vi "Point-in-Quad test (axis-aligned).vi"(1 "Point":sgl[](array[numeric]), 2 "Quad":T1) -> (0 "Point is inside quad":bool)   [LabVIEW 2014]
uses:
  Typedefs/Quad.ctl
  Typedefs/Quadplane enum.ctl
panel:
  # "PN 17/01/2015, 25/03/2015"
  # "Vertices"
  # "Edges"
  # "Unit normal"
  # "Plane ident."
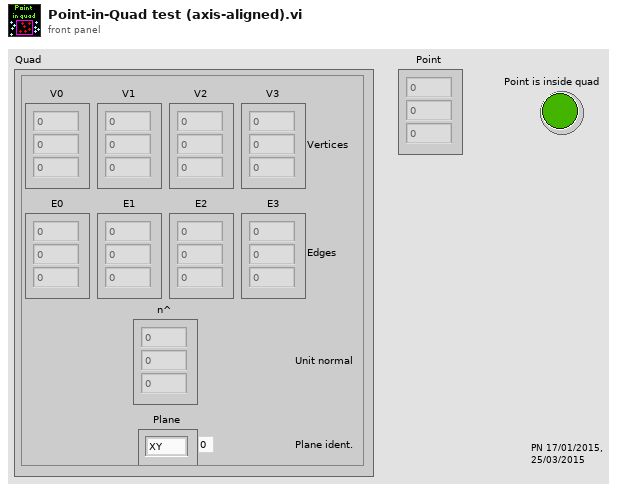
[diagram p1: front panel]
types:
  T1 = typedef "Quad.ctl" = cluster{"V0":sgl[], "V1":sgl[], "V2":sgl[], "V3":sgl[], "E0":sgl[], "E1":sgl[], "E2":sgl[], "E3":sgl[], "n^":sgl[], "Plane":T2}
  T2 = typedef "Quadplane enum.ctl" = enum8{"XY", "XZ", "YZ", "-XY", "-XZ", "-YZ"}
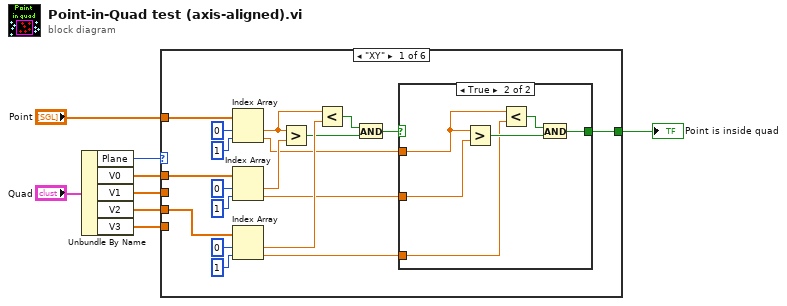
[diagram p0: block diagram]
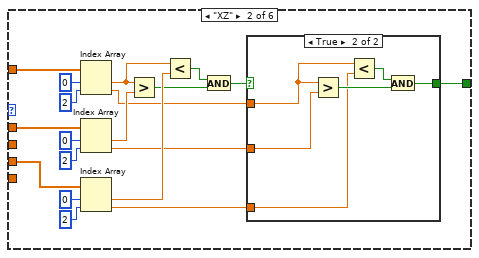
[diagram p3: hidden frame]
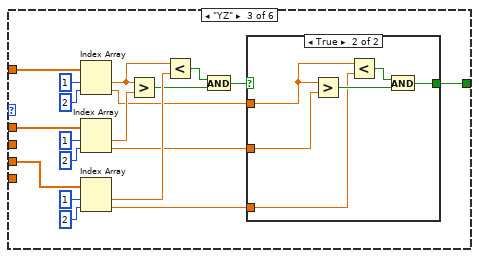
[diagram p5: hidden frame]
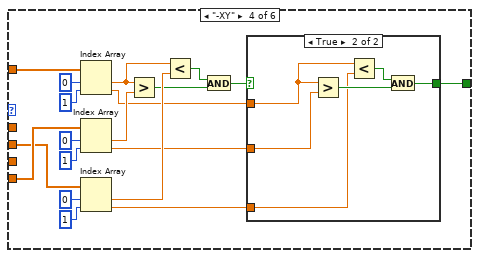
[diagram p7: hidden frame]
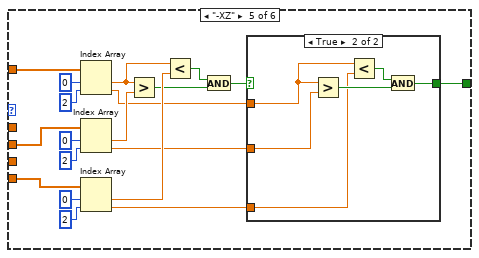
[diagram p9: hidden frame]
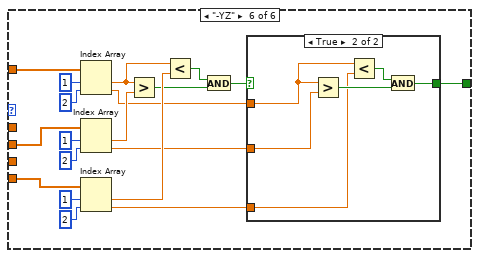
[diagram p11: hidden frame]
diagram:
  n1 = Unbundle By Name("Quad") -> ("Plane"=w7:T2, "V0"=w4:sgl[], "V1"=w2:sgl[], "V2"=w3:sgl[], "V3"=w1:sgl[])
  n2 = case shown="\"XY\"" w7 {
    tunnel: "Point" -> [w27 w53 w79 w105 w131 w157]
    tunnel: w3 -> [w25 w51 w77 _ _ _]
    tunnel: w4 -> [w26 w52 w78 _ _ _]
    tunnel: [w18 w44 w70 w98 w124 w150] -> w5
    tunnel: w2 -> [_ _ _ w87 w114 w140]
    tunnel: w1 -> [_ _ _ w88 w113 w139]
    frame "XY" {
      n3 = Index Array(array=w27, index #1=0 ("index"), index #2=1 ("index")) -> (element #1=w23:sgl, element #2=w17:sgl)
      n4 = Index Array(array=w26, index #1=0 ("index"), index #2=1 ("index")) -> (element #1=w24:sgl, element #2=w16:sgl)
      n5 = Index Array(array=w25, index #1=0 ("index"), index #2=1 ("index")) -> (element #1=w22:sgl, element #2=w15:sgl)
      n6 = Greater?(x=w23, y=w24) -> (0:w21:bool)
      n7 = Less?(x=w23, y=w22) -> (x < y?=w20:bool)
      n8 = And(x=w20, y=w21) -> (x .and. y?=w19:bool)
      n9 = case shown="True" w19 {
        selector: w19 -> [w28 _]
        tunnel: [w28 w32] -> w18
        tunnel: w17 -> [_ w30]
        tunnel: w16 -> [_ w31]
        tunnel: w15 -> [_ w29]
        frame False {
        }
        frame True {
          n10 = Greater?(x=w30, y=w31) -> (0:w33:bool)
          n11 = Less?(x=w30, y=w29) -> (x < y?=w34:bool)
          n12 = And(x=w34, y=w33) -> (x .and. y?=w32:bool)
        }
      }
    }
    frame "XZ" {
      n13 = Index Array(array=w53, index #1=0 ("index"), index #2=2 ("index")) -> (element #1=w49:sgl, element #2=w43:sgl)
      n14 = Index Array(array=w52, index #1=0 ("index"), index #2=2 ("index")) -> (element #1=w50:sgl, element #2=w42:sgl)
      n15 = Index Array(array=w51, index #1=0 ("index"), index #2=2 ("index")) -> (element #1=w48:sgl, element #2=w41:sgl)
      n16 = Greater?(x=w49, y=w50) -> (0:w47:bool)
      n17 = Less?(x=w49, y=w48) -> (x < y?=w46:bool)
      n18 = And(x=w46, y=w47) -> (x .and. y?=w45:bool)
      n19 = case shown="True" w45 {
        selector: w45 -> [w54 _]
        tunnel: [w54 w58] -> w44
        tunnel: w43 -> [_ w56]
        tunnel: w42 -> [_ w57]
        tunnel: w41 -> [_ w55]
        frame False {
        }
        frame True {
          n20 = Greater?(x=w56, y=w57) -> (0:w59:bool)
          n21 = Less?(x=w56, y=w55) -> (x < y?=w60:bool)
          n22 = And(x=w60, y=w59) -> (x .and. y?=w58:bool)
        }
      }
    }
    frame "YZ" {
      n23 = Index Array(array=w79, index #1=1 ("index"), index #2=2 ("index")) -> (element #1=w75:sgl, element #2=w69:sgl)
      n24 = Index Array(array=w78, index #1=1 ("index"), index #2=2 ("index")) -> (element #1=w76:sgl, element #2=w68:sgl)
      n25 = Index Array(array=w77, index #1=1 ("index"), index #2=2 ("index")) -> (element #1=w74:sgl, element #2=w67:sgl)
      n26 = Greater?(x=w75, y=w76) -> (0:w73:bool)
      n27 = Less?(x=w75, y=w74) -> (x < y?=w72:bool)
      n28 = And(x=w72, y=w73) -> (x .and. y?=w71:bool)
      n29 = case shown="True" w71 {
        selector: w71 -> [w80 _]
        tunnel: [w80 w84] -> w70
        tunnel: w69 -> [_ w82]
        tunnel: w68 -> [_ w83]
        tunnel: w67 -> [_ w81]
        frame False {
        }
        frame True {
          n30 = Greater?(x=w82, y=w83) -> (0:w85:bool)
          n31 = Less?(x=w82, y=w81) -> (x < y?=w86:bool)
          n32 = And(x=w86, y=w85) -> (x .and. y?=w84:bool)
        }
      }
    }
    frame "-XY" {
      n33 = Index Array(array=w105, index #1=0 ("index"), index #2=1 ("index")) -> (element #1=w103:sgl, element #2=w97:sgl)
      n34 = Index Array(array=w88, index #1=0 ("index"), index #2=1 ("index")) -> (element #1=w104:sgl, element #2=w96:sgl)
      n35 = Index Array(array=w87, index #1=0 ("index"), index #2=1 ("index")) -> (element #1=w102:sgl, element #2=w95:sgl)
      n36 = Greater?(x=w103, y=w104) -> (0:w101:bool)
      n37 = Less?(x=w103, y=w102) -> (x < y?=w100:bool)
      n38 = And(x=w100, y=w101) -> (x .and. y?=w99:bool)
      n39 = case shown="True" w99 {
        selector: w99 -> [w106 _]
        tunnel: [w106 w110] -> w98
        tunnel: w97 -> [_ w108]
        tunnel: w96 -> [_ w109]
        tunnel: w95 -> [_ w107]
        frame False {
        }
        frame True {
          n40 = Greater?(x=w108, y=w109) -> (0:w111:bool)
          n41 = Less?(x=w108, y=w107) -> (x < y?=w112:bool)
          n42 = And(x=w112, y=w111) -> (x .and. y?=w110:bool)
        }
      }
    }
    frame "-XZ" {
      n43 = Index Array(array=w131, index #1=0 ("index"), index #2=2 ("index")) -> (element #1=w129:sgl, element #2=w123:sgl)
      n44 = Index Array(array=w114, index #1=0 ("index"), index #2=2 ("index")) -> (element #1=w130:sgl, element #2=w122:sgl)
      n45 = Index Array(array=w113, index #1=0 ("index"), index #2=2 ("index")) -> (element #1=w128:sgl, element #2=w121:sgl)
      n46 = Greater?(x=w129, y=w130) -> (0:w127:bool)
      n47 = Less?(x=w129, y=w128) -> (x < y?=w126:bool)
      n48 = And(x=w126, y=w127) -> (x .and. y?=w125:bool)
      n49 = case shown="True" w125 {
        selector: w125 -> [w132 _]
        tunnel: [w132 w136] -> w124
        tunnel: w123 -> [_ w134]
        tunnel: w122 -> [_ w135]
        tunnel: w121 -> [_ w133]
        frame False {
        }
        frame True {
          n50 = Greater?(x=w134, y=w135) -> (0:w137:bool)
          n51 = Less?(x=w134, y=w133) -> (x < y?=w138:bool)
          n52 = And(x=w138, y=w137) -> (x .and. y?=w136:bool)
        }
      }
    }
    frame "-YZ" {
      n53 = Index Array(array=w157, index #1=1 ("index"), index #2=2 ("index")) -> (element #1=w155:sgl, element #2=w149:sgl)
      n54 = Index Array(array=w140, index #1=1 ("index"), index #2=2 ("index")) -> (element #1=w156:sgl, element #2=w148:sgl)
      n55 = Index Array(array=w139, index #1=1 ("index"), index #2=2 ("index")) -> (element #1=w154:sgl, element #2=w147:sgl)
      n56 = Greater?(x=w155, y=w156) -> (0:w153:bool)
      n57 = Less?(x=w155, y=w154) -> (x < y?=w152:bool)
      n58 = And(x=w152, y=w153) -> (x .and. y?=w151:bool)
      n59 = case shown="True" w151 {
        selector: w151 -> [w158 _]
        tunnel: [w158 w162] -> w150
        tunnel: w149 -> [_ w160]
        tunnel: w148 -> [_ w161]
        tunnel: w147 -> [_ w159]
        frame False {
        }
        frame True {
          n60 = Greater?(x=w160, y=w161) -> (0:w163:bool)
          n61 = Less?(x=w160, y=w159) -> (x < y?=w164:bool)
          n62 = And(x=w164, y=w163) -> (x .and. y?=w162:bool)
        }
      }
    }
  }
  "Point is inside quad" <- w5
